vi "Change Calibration State.vi"(8 "error in":errorcluster, 10 "New State":bool, 11 "Calibration UI in":refnum<class "Calibration UI.lvclass">) -> (0 "error out":errorcluster, 3 "Calibration UI out":refnum<class "Calibration UI.lvclass">)   [LabVIEW 2015, in "Calibration UI.lvclass"]
uses:
  Calibration UI.lvclass
  Calibration UI.lvclass/Calibration UI.ctl
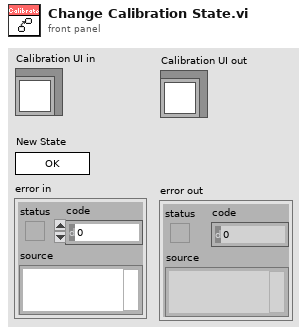
[diagram p1: front panel]
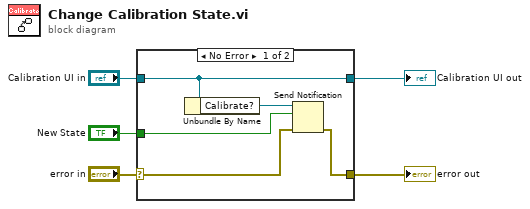
[diagram p0: block diagram]
diagram:
  n1 = case shown="No Error" "error in" {
    selector: "error in" -> [w7 w12]
    tunnel: [w6 w12] -> w4
    tunnel: [w10 w11] -> w2
    tunnel: "Calibration UI in" -> [w10 w11]
    tunnel: "New State" -> [w8 _]
    frame No Error {
      n2 = Unbundle By Name(w10) -> ("Calibrate?"=w9:refnum<notifier>)
      n3 = Send Notification(notification=w8, notifier=w9, error in (no error)=w7) -> (error out=w6:errorcluster)  [unwired: 1 out]
    }
    frame Error {
    }
  }
  "error out" <- w4
  "Calibration UI out" <- w2
